vi "Create Client.vi"(8 "error in":errorcluster) -> (0 "error out":errorcluster, 3 "grpc client id":T1)   [LabVIEW 2020, in "MeasurementLink Discovery.lvlib"]
uses:
  MeasurementLink Discovery.lvlib
  <vilib>/gRPC/LabVIEW gRPC Library/Shared/grpcId.ctl
  MeasurementLink Measurement Server/MeasurementLink Measurement Server.lvlib
  MeasurementLink Discovery Client/MeasurementLink Discovery Client.lvlib
  <vilib>/gRPC/LabVIEW gRPC Library/grpc-lvsupport-release.lvlib
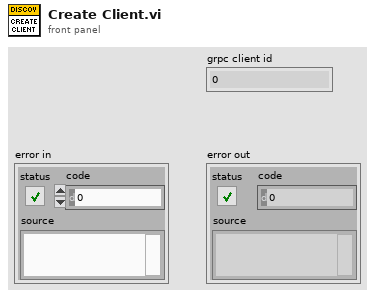
[diagram p1: front panel]
types:
  T1 = typedef "grpc-lvsupport-release.lvlib/grpcId.ctl" = u64
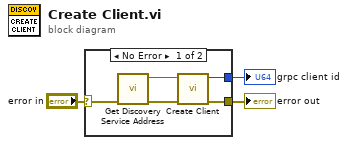
[diagram p0: block diagram]
diagram:
  n1 = case shown="No Error" "error in" {
    selector: "error in" -> [w6 w9]
    tunnel: [w8 _] -> w3
    tunnel: [w7 w9] -> w2
    frame No Error {
      n2 = call "Get Discovery Service Address.vi"("error in"=w6) -> ("error out"=w4:errorcluster, "address"=w5:string)  [unwired: 9 in]
      n3 = call "Create Client.vi"("error in"=w4, "address"=w5) -> ("error out"=w7:errorcluster, "gRPC ID Out"=w8:T1)  [unwired: 8 in]
    }
    frame Error {
    }
  }
  "grpc client id" <- w3
  "error out" <- w2
